vi "FPGA Main.vi"() -> ()   [LabVIEW 2012]
doc: "This FPGA Main VI contains a control loop running in parallel with an RT watchdog loop.\n- The Control Loop performs control calculations on four input channels in parallel, and outputs the results to four output channels.\n- The RT Watchdog Loop checks for a periodic 'pet' from the RT Main VI to ensure communications between RT and FPGA are maintained."
uses:
  controls/FPGA State.ctl
  controls/Control Configuration.ctl
  controls/Raw Values.ctl
  <vilib>/rvi/Emulation/niFpgaSctlEmulationGetInTimedLoop.vi
  <vilib>/rvi/Emulation/niFpgaSctlEmulationGlobalWrite.vi
  <vilib>/rvi/eio/common/nirviEmuTemplateMethod_errors.vi
  <vilib>/eio/EIONode/EIONode.xnode
panel:
  in  "Channel 3 Setpoint":fxp<+/-,16,5>
  in  "Channel 2 Setpoint":fxp<+/-,16,5>
  in  "Channel 1 Setpoint":fxp<+/-,16,5>
  in  "Channel 0 Setpoint":fxp<+/-,16,5>
  out "Watchdog Timed Out?":bool=TRUE
  in  "Enable Watchdog":bool
  in  "Pet Watchdog":bool
  in  "Watchdog Timeout Period (ticks)":u64=40000000 format="%.0p"
  out "Time Since Last Pet":u64
  in  "Manual Values":T1
  out "Output Values":T1
  out "Input Values":T1
  in  "Channel 3 Configuration":T2={"PID Gains"={"proportional gain (Kc)"=0.0, "integral gain (Kc*Ts/Ti)"=0.0, "derivative gain (Kc*Td/Ts)"=0.0}, "Output Range"={"output high"=10.0, "output low"=-10.0}}
  in  "Channel 2 Configuration":T2={"PID Gains"={"proportional gain (Kc)"=0.0, "integral gain (Kc*Ts/Ti)"=0.0, "derivative gain (Kc*Td/Ts)"=0.0}, "Output Range"={"output high"=10.0, "output low"=-10.0}}
  in  "Channel 1 Configuration":T2={"PID Gains"={"proportional gain (Kc)"=0.0, "integral gain (Kc*Ts/Ti)"=0.0, "derivative gain (Kc*Td/Ts)"=0.0}, "Output Range"={"output high"=10.0, "output low"=-10.0}}
  in  "Channel 0 Configuration":T2={"PID Gains"={"proportional gain (Kc)"=0.0, "integral gain (Kc*Ts/Ti)"=0.0, "derivative gain (Kc*Td/Ts)"=0.0}, "Output Range"={"output high"=10.0, "output low"=-10.0}}
  in  "New State":T3=enum."Control (PID)"
  out "Actual Loop Period (ticks)":u32
  out "Current FPGA State":T3=enum."Manual"
  in  "Change State":bool
  out "Input Error":bool
  out "Output Error":bool
  in  "Control Period (ticks)":u32
  # "General Settings"
  # "Manual Settings"
  # "Monitoring Values"
  # "Watchdog Settings"
  # "Control Settings"
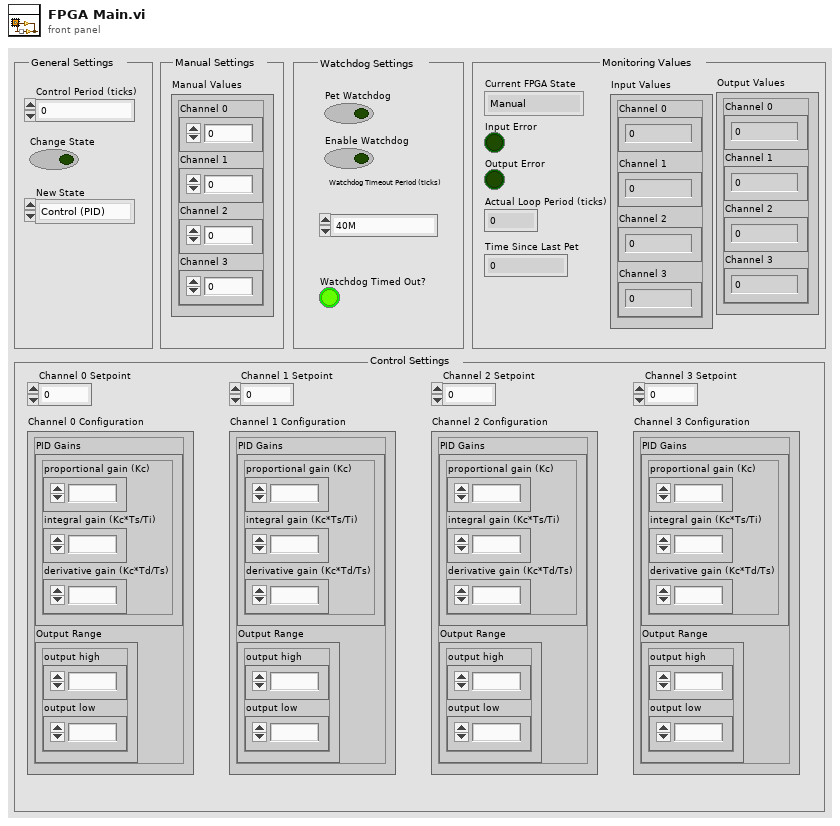
[diagram p1: front panel]
types:
  T1 = typedef "Raw Values.ctl" = cluster{"Channel 0":fxp<+/-,20,5>, "Channel 1":fxp<+/-,20,5>, "Channel 2":fxp<+/-,20,5>, "Channel 3":fxp<+/-,20,5>}
  T2 = typedef "Control Configuration.ctl" = cluster{"PID Gains":cluster{"proportional gain (Kc)":fxp<+/-,16,8>, "integral gain (Kc*Ts/Ti)":fxp<+/-,16,8>, "derivative gain (Kc*Td/Ts)":fxp<+/-,16,8>}, "Output Range":cluster{"output high":fxp<+/-,16,5>, "output low":fxp<+/-,16,5>}}
  T3 = typedef "FPGA State.ctl" = enum16{"Safe State", "Manual", "Control (PID)"}
  T4 = cluster{"proportional gain (Kc)":fxp<+/-,16,8>, "integral gain (Kc*Ts/Ti)":fxp<+/-,16,8>, "derivative gain (Kc*Td/Ts)":fxp<+/-,16,8>}
  T5 = cluster{"output high":fxp<+/-,16,5>, "output low":fxp<+/-,16,5>}
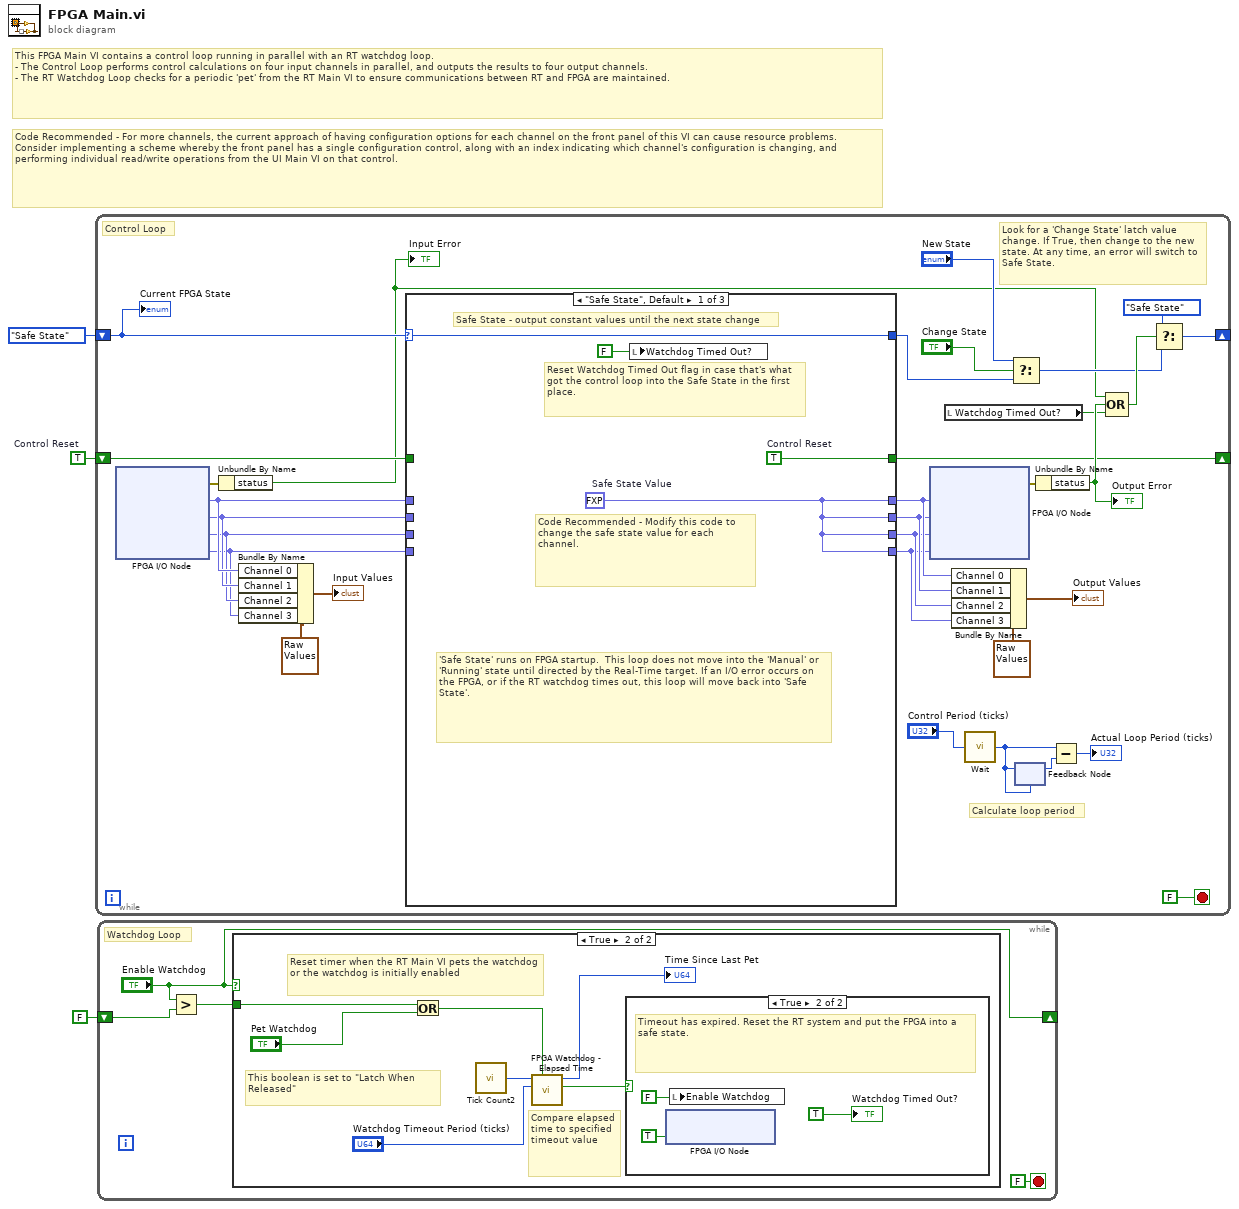
[diagram p0: block diagram]
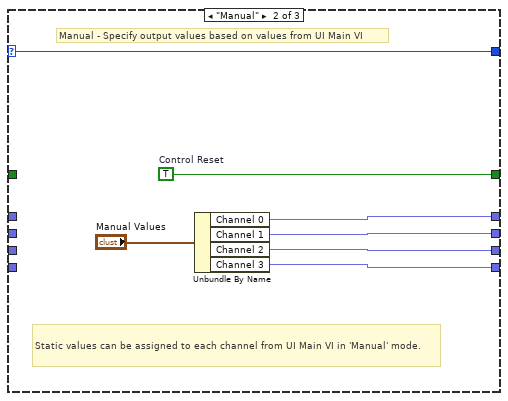
[diagram p4: hidden frame]
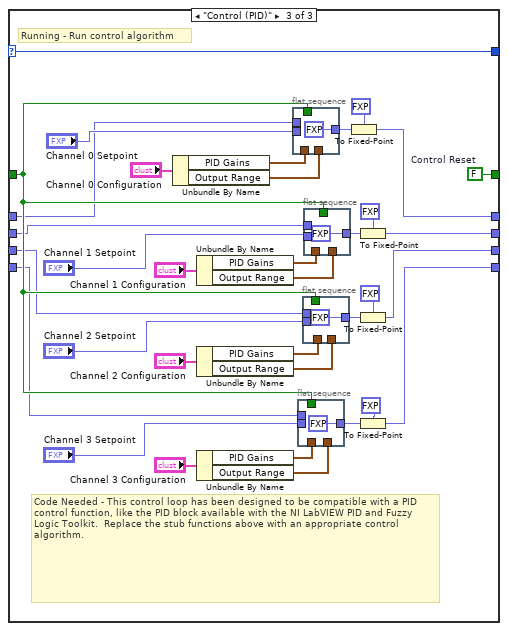
[diagram p5: hidden frame]
diagram:
  w2 = TRUE  # Control Reset
  # "Code Recommended - For more channels, the current approach of having configuration options for each channel on the front panel of this VI can cause resource problems.  Consider implementing a scheme whereby the front panel has a single configuration control, along with an index indicating which channel's configuration is changing, and performing individual read/write operations from the UI Main VI on that control."
  # "This FPGA Main VI contains a control loop running in parallel with an RT watchdog loop.\n- The Control Loop performs control calculations on four input channels in parallel, and outputs the results to four output channels.\n- The RT Watchdog Loop checks for a periodic 'pet' from the RT Main VI to ensure communications between RT and FPGA are maintained."
  n1 = while {
    shift-right: [w30] -> _
    shift-left: FPGA_State."Safe State" ("FPGA State") -> [w21]
    shift-right: [w27] -> _
    shift-left: w2 -> [w26]
    stop <- FALSE stop-if-true
    # "Calculate loop period"
    # "Look for a 'Change State' latch value change. If True, then change to the new state. At any time, an error will switch to Safe State."
    # "Control Loop"
    n2 = xnode "FPGA I/O Node"() -> ("error out"=w34:errorcluster, "Mod1/AI0"=w19:fxp<+/-,16,5>, "Mod1/AI1"=w18:fxp<+/-,16,5>, "Mod1/AI2"=w17:fxp<+/-,16,5>, "Mod1/AI3"=w16:fxp<+/-,16,5>)  [unwired: 5 in, 4 out]
    n3 = Unbundle By Name(w34) -> ("status"=w20:bool)
    "Input Error" <- w20
    n4 = Bundle By Name(cluster=T1 {"Channel 0"=0.0, "Channel 1"=0.0, "Channel 2"=0.0, "Channel 3"=0.0} ("Raw Values"), "Channel 0"=w19, "Channel 1"=w18, "Channel 2"=w17, "Channel 3"=w16) -> (→"Input Values":T1)
    n5 = case shown="\"Safe State\", Default" w21 {
      selector: w21 -> [w38 w45 w78]
      tunnel: w19 -> [_ _ w51]
      tunnel: [w37 w43 w80] -> w15
      tunnel: [w38 w45 w78] -> w25
      tunnel: [w39 w46 w79] -> w27
      tunnel: w26 -> [_ _ w55]
      tunnel: w18 -> [_ _ w52]
      tunnel: w17 -> [_ _ w53]
      tunnel: w16 -> [_ _ w54]
      tunnel: [w37 w42 w70] -> w14
      tunnel: [w37 w41 w69] -> w13
      tunnel: [w37 w40 w68] -> w12
      frame "Safe State", Default {
        w37 = fxp<+/-,20,5> 0.0  # Safe State Value
        w39 = TRUE  # Control Reset
        # "'Safe State' runs on FPGA startup.  This loop does not move into the 'Manual' or 'Running' state until directed by the Real-Time target. If an I/O error occurs on the FPGA, or if the RT watchdog times out, this loop will move back into 'Safe State'."
        # "Reset Watchdog Timed Out flag in case that's what got the control loop into the Safe State in the first place."
        # "Safe State - output constant values until the next state change"
        # "Code Recommended - Modify this code to change the safe state value for each channel."
        n6 = local write "Watchdog Timed Out?"(FALSE ("Watchdog Timed Out?")) -> ()
      }
      frame "Manual" {
        w46 = TRUE  # Control Reset
        # "Manual - Specify output values based on values from UI Main VI"
        # "Static values can be assigned to each channel from UI Main VI in 'Manual' mode."
        n7 = Unbundle By Name("Manual Values") -> ("Channel 0"=w43:fxp<+/-,20,5>, "Channel 1"=w42:fxp<+/-,20,5>, "Channel 2"=w41:fxp<+/-,20,5>, "Channel 3"=w40:fxp<+/-,20,5>)
      }
      frame "Control (PID)" {
        w79 = FALSE  # Control Reset
        # "Running - Run control algorithm"
        # "Code Needed - This control loop has been designed to be compatible with a PID control function, like the PID block available with the NI LabVIEW PID and Fuzzy Logic Toolkit.  Replace the stub functions above with an appropriate control algorithm."
        n8 = Unbundle By Name("Channel 0 Configuration") -> ("PID Gains"=w58:T4, "Output Range"=w57:T5)
        n9 = Unbundle By Name("Channel 1 Configuration") -> ("PID Gains"=w61:T4, "Output Range"=w60:T5)
        n10 = Unbundle By Name("Channel 2 Configuration") -> ("PID Gains"=w64:T4, "Output Range"=w63:T5)
        n11 = Unbundle By Name("Channel 3 Configuration") -> ("PID Gains"=w67:T4, "Output Range"=w66:T5)
        n12 = flat-sequence {
          tunnel: w58 -> [_]
          tunnel: w57 -> [_]
          tunnel: "Channel 0 Setpoint" -> [_]
          tunnel: w55 -> [_]
          tunnel: w51 -> [_]
          tunnel: [fxp<+/-,16,5> 0.0 ("output")] -> w47
          frame #0 {
          }
        }
        n13 = flat-sequence {
          tunnel: w67 -> [_]
          tunnel: w66 -> [_]
          tunnel: "Channel 3 Setpoint" -> [_]
          tunnel: w55 -> [_]
          tunnel: w54 -> [_]
          tunnel: [fxp<+/-,16,5> 0.0 ("output")] -> w50
          frame #0 {
          }
        }
        n14 = flat-sequence {
          tunnel: w64 -> [_]
          tunnel: w63 -> [_]
          tunnel: "Channel 2 Setpoint" -> [_]
          tunnel: w55 -> [_]
          tunnel: w53 -> [_]
          tunnel: [fxp<+/-,16,5> 0.0 ("output")] -> w49
          frame #0 {
          }
        }
        n15 = flat-sequence {
          tunnel: w61 -> [_]
          tunnel: w60 -> [_]
          tunnel: "Channel 1 Setpoint" -> [_]
          tunnel: w55 -> [_]
          tunnel: w52 -> [_]
          tunnel: [fxp<+/-,16,5> 0.0 ("output")] -> w48
          frame #0 {
          }
        }
        n16 = To Fixed-Point(fixed-point type=fxp<+/-,20,5> 0.0 ("Off Value"), number=w47) -> (fixed-point=w80:fxp<+/-,20,5>)
        n17 = To Fixed-Point(fixed-point type=fxp<+/-,20,5> 0.0 ("Off Value"), number=w48) -> (fixed-point=w70:fxp<+/-,20,5>)
        n18 = To Fixed-Point(fixed-point type=fxp<+/-,20,5> 0.0 ("Off Value"), number=w49) -> (fixed-point=w69:fxp<+/-,20,5>)
        n19 = To Fixed-Point(fixed-point type=fxp<+/-,20,5> 0.0 ("Off Value"), number=w50) -> (fixed-point=w68:fxp<+/-,20,5>)
      }
    }
    n20 = xnode "FPGA I/O Node"("Mod2/AO0"=w15, "Mod2/AO1"=w14, "Mod2/AO2"=w13, "Mod2/AO3"=w12) -> ("error out"=w33:errorcluster)  [unwired: 5 in, 4 out]
    n21 = local read "Watchdog Timed Out?"() -> (w9:bool)
    n22 = Bundle By Name(cluster=T1 {"Channel 0"=0.0, "Channel 1"=0.0, "Channel 2"=0.0, "Channel 3"=0.0} ("Raw Values"), "Channel 0"=w15, "Channel 1"=w14, "Channel 2"=w13, "Channel 3"=w12) -> (→"Output Values":T1)
    n23 = call "Wait"("Count(Ticks)"="Control Period (ticks)") -> ("Tick Count(Ticks)"=w8:u32)
    n24 = Select(t="New State", s="Change State", f=w25) -> (s? t:f=w22:T3)
    n25 = feedback-in #1(w8) -> ()
    n26 = feedback #1(w8) -> (w7:u32)
    n27 = Unbundle By Name(w33) -> ("status"=w32:bool)
    "Output Error" <- w32
    n28 = Subtract(x=w8, y=w7) -> (x-y=→"Actual Loop Period (ticks)":u32)
    n29 = Compound Arithmetic op=OR(w20, w32, w9) -> (w29:bool)
    n30 = Select(t=FPGA_State."Safe State" ("FPGA State"), s=w29, f=w22) -> (s? t:f=w30:T3)
    "Current FPGA State" <- w21
  }
  n31 = while "RT Watchdog Loop" {
    shift-right: ["Enable Watchdog"] -> _
    shift-left: FALSE ("Enable RT Watchdog") -> [w89]
    stop <- FALSE stop-if-true
    # "Watchdog Loop"
    n32 = Greater?(x="Enable Watchdog", y=w89) -> (0:w86:bool)
    n33 = case shown="True" "Enable Watchdog" {
      tunnel: w86 -> [_ w92]
      frame False {
        # "This loop has to be explicitly enabled from the RT Main VI.  This reduces the possiblity of an endless reboot cycle."
      }
      frame True {
        # "This boolean is set to \"Latch When Released\""
        # "Compare elapsed time to specified timeout value"
        # "Reset timer when the RT Main VI pets the watchdog or the watchdog is initially enabled"
        n34 = Or(x=w92, y="Pet Watchdog") -> (x .or. y?=w91:bool)
        n35 = call "Tick Count2"() -> ("Tick Count(Ticks)"=w95:u32)
        n36 = call "FPGA Watchdog - Elapsed Time.vi"("Reset"=w91, "Timeout Period"="Watchdog Timeout Period (ticks)", "Current Time"=w95) -> ("Timeout"=w90:bool, "Elapsed Time"=→"Time Since Last Pet":u64)  [unwired: 7 in]
        n37 = case shown="True" w90 {
          frame False {
            # "Timeout has not expired."
          }
          frame True {
            # "Timeout has expired. Reset the RT system and put the FPGA into a safe state."
            n38 = xnode "FPGA I/O Node"("System Reset"=TRUE ("RT Reset on Watchdog Failure?")) -> ()  [unwired: 1 in, 1 out]
            n39 = local write "Enable Watchdog"(FALSE ("Enable RT Watchdog")) -> ()
            "Watchdog Timed Out?" <- TRUE ("Watchdog Timed Out?")
          }
        }
      }
    }
  }
